vi "Setup Turbo Valve Settings.vi"(8 "error in (no error)":errorcluster, 10 "Model in":refnum<class "Model.lvclass">, 11 "Boot Loader in":refnum<class "Boot Loader.lvclass">) -> (0 "error out":errorcluster, 2 "Model out":refnum<class "Model.lvclass">, 3 "Boot Loader out":refnum<class "Boot Loader.lvclass">)   [LabVIEW 2015, in "Boot Loader.lvclass"]
uses:
  Boot Loader.lvclass
  Model/Model.lvclass
  Model/Model.lvclass/Model.ctl
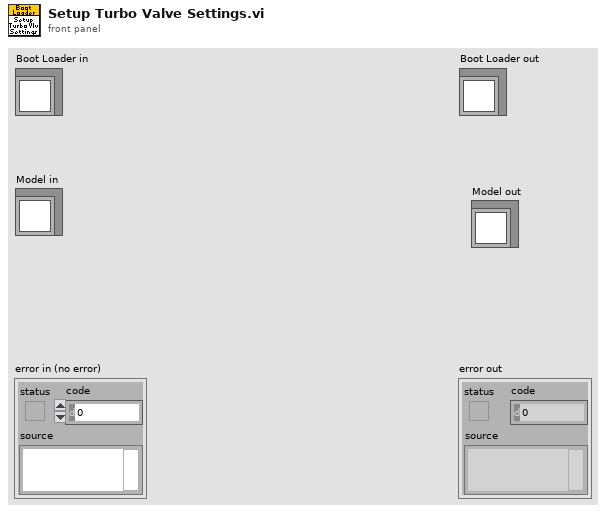
[diagram p1: front panel]
types:
  T1 = typedef "FAMT Typedefs.lvlib/Turbo Valve Settings.ctl" = cluster{"ROT Bias":u8, "Minimum Voltage":dbl, "Maximum Voltage":dbl, "Off Value":dbl}
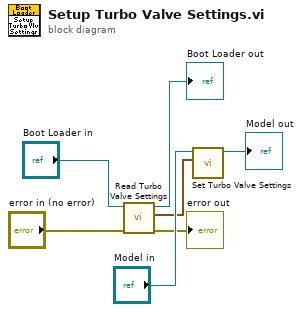
[diagram p0: block diagram]
diagram:
  n1 = call "Read Turbo Valve Settings.vi"("error in (no error)"="error in (no error)", "Boot Loader in"="Boot Loader in") -> ("error out"=→"error out":errorcluster, "Turbo Valve Settings"=w1:T1, "Boot Loader out"=→"Boot Loader out":refnum<class "Boot Loader.lvclass">)  [unwired: 7 in]
  n2 = call "Set Turbo Valve Settings.vi"("Turbo Valve Settings"=w1, "Model in"="Model in") -> ("Model out"=→"Model out":refnum<class "Model.lvclass">)  [unwired: 9 in]
